vi "dealWithWeek.vi"(8 "初始日":i32=1, 9 "input_day":i32=1, 10 "input_firstWeek":i32, 11 "input_week":i32) -> (3 "ddd":i32)   [LabVIEW 2011]
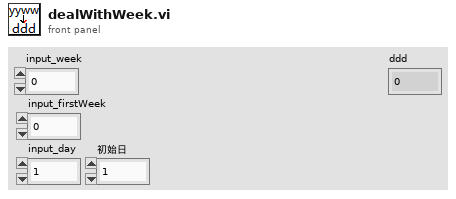
[diagram p1: front panel]
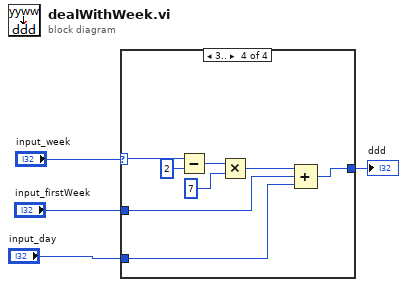
[diagram p0: block diagram]
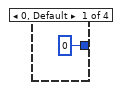
[diagram p2: hidden frame]
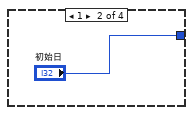
[diagram p3: hidden frame]
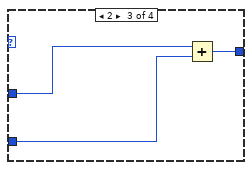
[diagram p4: hidden frame]
diagram:
  n1 = case shown="3.." "input_week" {
    selector: "input_week" -> [_ _ _ w14]
    tunnel: [0 ("input_firstWeek") "初始日" w9 w11] -> w2
    tunnel: "input_firstWeek" -> [_ _ w8 w12]
    tunnel: "input_day" -> [_ _ w7 w10]
    frame 0, Default {
    }
    frame 1 {
    }
    frame 2 {
      n2 = Add(x=w8, y=w7) -> (x+y=w9:i32)
    }
    frame 3.. {
      n3 = Subtract(x=w14, y=2) -> (x-y=w17:i32)
      n4 = Multiply(x=w17, y=7) -> (x*y=w13:i32)
      n5 = Compound Arithmetic op=ADD(w13, w12, w10) -> (w11:i32)
    }
  }
  "ddd" <- w2
